vi "Broadcast TCU Settings.vi"(8 "error in (no error)":errorcluster, 10 "Message Queues":T9, 11 "Pump Module Config":T1={"GUID"="", "Drop Coords"={"Horizontal"=0, "Vertical"=0}, "Process Name"="", "Settings"={"Cycle Period"=500.0, "Setpoint Entry"=0.0, "Output Device"=enum."Default", "Huber Ministat 230 Settings"={"VISA resource name"="", "Simulated?"=TRUE}, "Lauda Settings"={"VISA resource name"="", "Simulated?"=FALSE, "Pump Power"=2}, "Julabo FP-50 Settings"={"VISA resource name"="", "Simulated?"=FALSE, "Pump Power"=2}, "Internal Control?"=FALSE, "Huber Unistat 410 Settings"={"VISA resource name"="", "Simulated?"=FALSE}}, "Load Count"=0, "Power Level Changed"=FALSE} {"Settings"."Julabo FP-50 Settings"."Pump Power" min=0 max=8 step=1; "Settings"."Lauda Settings"."Pump Power" min=0 max=8 step=1}) -> (0 "error out":errorcluster)   [LabVIEW 2018, in "TCU Module.lvlib"]
uses:
  TCU Module.lvlib
  All Message Queues.ctl
  support/Message Queue/Message Cluster.ctl
  TCU Module Config Cluster.ctl
  <vilib>/Utility/miscctls.llb/LVPoint32TypeDef.ctl
  TCU Module Settings Cluster.ctl
  Measure Instrument/Output Devices.ctl
  Huber TCU/Huber Settings.ctl
  Lauda Integral XT-150 TCU/Lauda Settings.ctl
  Julabo Type 1 TCU/Julabo Type 1 TCU Folder/Julabo FP-50 Settings.ctl
  Huber Unistat 410 TCU/Huber Unistat 410 Settings.ctl
  support/Message Queue/Enqueue Message (Single).vi
  support/Message Queue/Message Queue.lvlib
  Shared Variables/Dynamic Shared Variables.lvlib
  Huber TCU/Huber Ministat 230 TCU.lvlib
  Lauda Integral XT-150 TCU/Lauda TCU.lvlib
  Julabo Type 1 TCU/Julabo Type 1 TCU Folder/Julabo Type FP-50 TCU.lvlib
  Huber Unistat 410 TCU/Huber Unistat 410 TCU.lvlib
panel:
  # "Output Instruments"
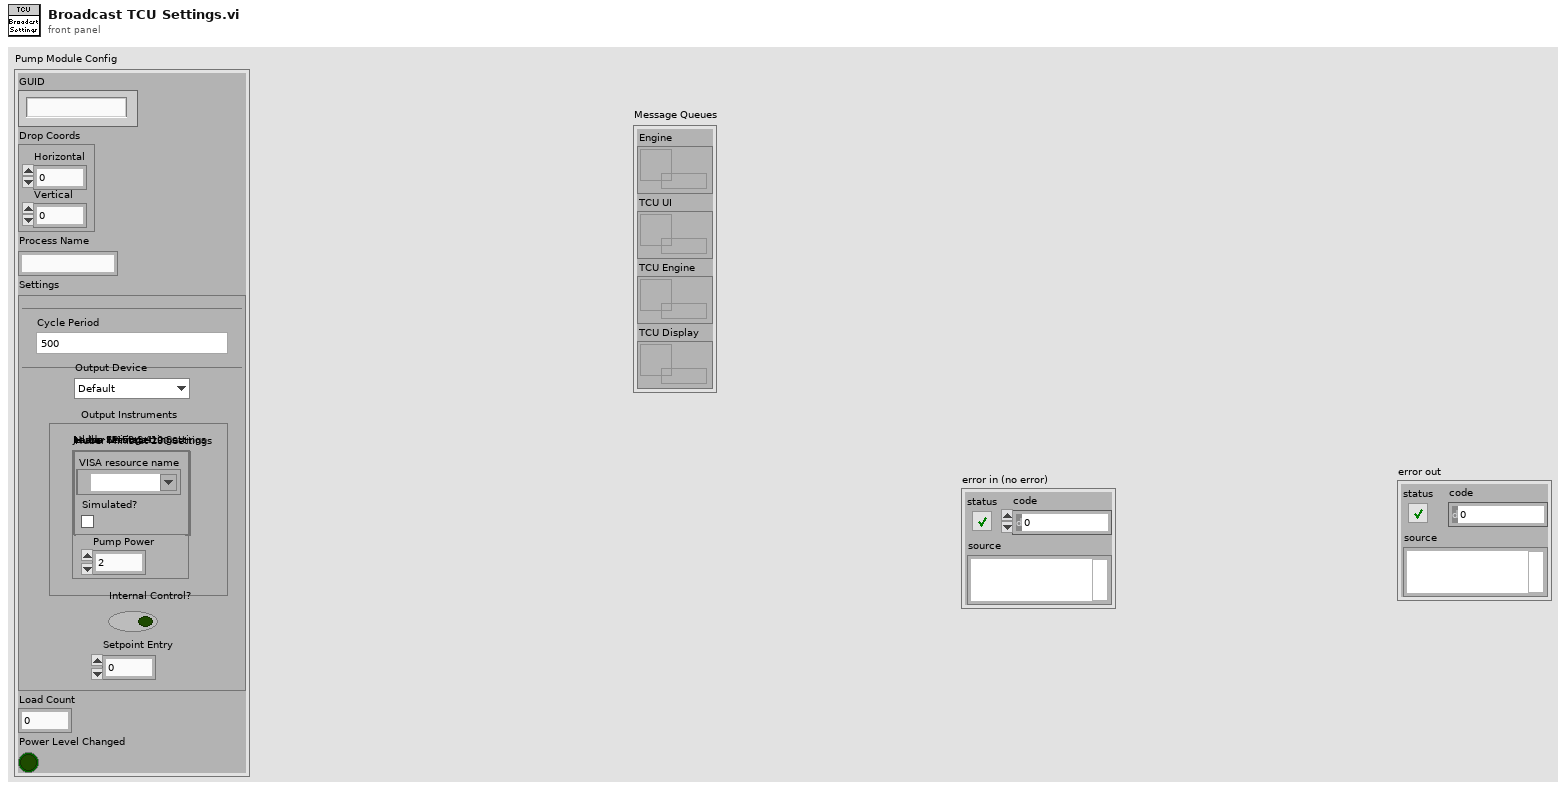
[diagram p1: front panel]
types:
  T1 = typedef "TCU Module.lvlib/TCU Module Config Cluster.ctl" = cluster{"GUID":string, "Drop Coords":T2, "Process Name":string, "Settings":T3, "Load Count":i32, "Power Level Changed":bool}
  T2 = typedef "LVPoint32TypeDef.ctl" = cluster{"Horizontal":i32, "Vertical":i32}
  T3 = typedef "TCU Module.lvlib/TCU Module Settings Cluster.ctl" = cluster{"Cycle Period":dbl, "Setpoint Entry":dbl, "Output Device":T4, "Huber Ministat 230 Settings":T5, "Lauda Settings":T6, "Julabo FP-50 Settings":T7, "Internal Control?":bool, "Huber Unistat 410 Settings":T8}
  T4 = typedef "Output Devices.ctl" = enum16{"Default", "Huber Ministat 230", "Huber Unistat 410", "Lauda XT-150", "Julabo FP-50"}
  T5 = typedef "Huber Ministat 230 TCU.lvlib/Huber Settings.ctl" = cluster{"VISA resource name":refnum<visa-resource-name>, "Simulated?":bool}
  T6 = typedef "Lauda TCU.lvlib/Lauda Settings.ctl" = cluster{"VISA resource name":refnum<visa-resource-name>, "Simulated?":bool, "Pump Power":i32}
  T7 = typedef "Julabo Type FP-50 TCU.lvlib/Julabo FP-50 Settings.ctl" = cluster{"VISA resource name":refnum<visa-resource-name>, "Simulated?":bool, "Pump Power":i32}
  T8 = typedef "Huber Unistat 410 TCU.lvlib/Huber Unistat 410 Settings.ctl" = cluster{"VISA resource name":refnum<visa-resource-name>, "Simulated?":bool}
  T9 = typedef "TCU Module.lvlib/All Message Queues.ctl" = cluster{"Engine":refnum<queue>, "TCU UI":refnum<queue>, "TCU Engine":refnum<queue>, "TCU Display":refnum<queue>}
  T10 = cluster{"enable? (F)":bool, "name":string, "alarm on":bool, "priority":u32, "ack type":enum16{"Auto", "User", "None", "Each Occurrence"}, "area":string, "description":string, "log? (T)":bool}
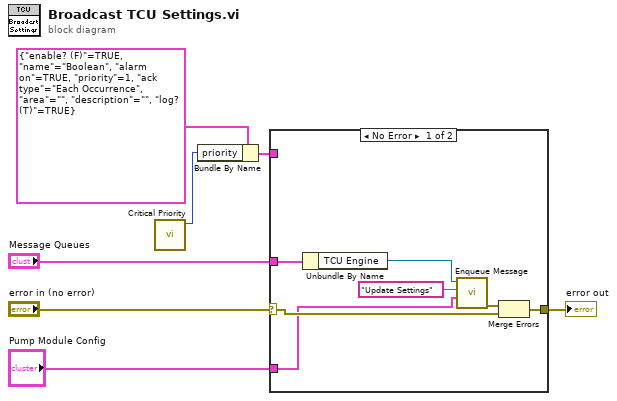
[diagram p0: block diagram]
diagram:
  n1 = call "Critical Priority.vi"() -> ("critical priority"=w3:i32)  [unwired: 11 in]
  n2 = Bundle By Name(cluster=T10 {"enable? (F)"=TRUE, "name"="Boolean", "alarm on"=TRUE, "priority"=1, "ack type"=enum."Each Occurrence", "area"="", "description"="", "log? (T)"=TRUE} ("Boolean alarm settings"), "priority"=w3) -> (w2:T10)
  n3 = case shown="No Error" "error in (no error)" {
    selector: "error in (no error)" -> [w13 w15]
    tunnel: [w14 w15] -> w5
    tunnel: "Pump Module Config" -> [w8 _]
    tunnel: "Message Queues" -> [w12 _]
    tunnel: w2 -> [_ _]
    frame No Error {
      n4 = Unbundle By Name(w12) -> ("TCU Engine"=w11:refnum<queue>)
      n5 = call-poly "Enqueue Message.vi"("Message Data"=w8, "Message"="Update Settings", "Message Queue"=w11) -> ("error out"=w10:errorcluster)  [unwired: 7 in, 1 out]
      n6 = Merge Errors(w10, w13) -> (w14:errorcluster)
    }
    frame Error {
    }
  }
  "error out" <- w5
